vi "Double to U16 Array.vi"(10 "Double":dbl) -> (2 "U16 Array":u16[](array[numeric]))   [LabVIEW 2015, in "Modbus Data Conversion.lvlib"]
uses:
  Modbus Data Conversion.lvlib
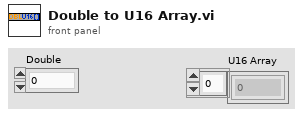
[diagram p1: front panel]
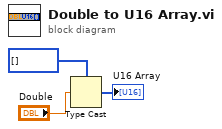
[diagram p0: block diagram]
diagram:
  n1 = Type Cast(type=u16[] [] ("U16 Array"), x="Double") -> (*(type *) &x=→"U16 Array":u16[])
